vi "Count Itteration.vi"(1 "Reset":bool, 2 "Enable":bool=TRUE, 3 "Direction (Up)":bool=TRUE) -> (4 "Itterations/s":dbl, 7 "Itteration":i32)   [LabVIEW 2012]
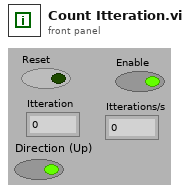
[diagram p1: front panel]
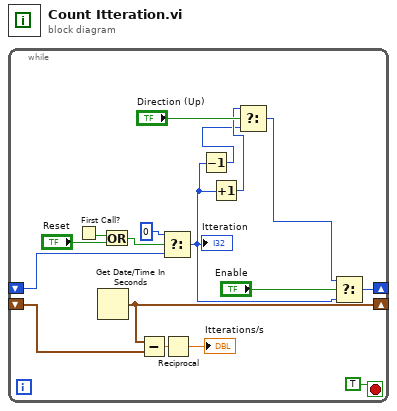
[diagram p0: block diagram]
diagram:
  n1 = while {
    shift-right: [w10] -> _
    shift-left: _ -> [w14]
    shift-right: [w7] -> _
    shift-left: _ -> [w8]
    stop <- TRUE stop-if-true
    n2 = First Call?() -> (First Call?: T/F=w16:bool)
    n3 = Get Date/Time In Seconds() -> (seconds since 1Jan1904=w7:timestamp)
    n4 = Or(x=w16, y="Reset") -> (x .or. y?=w12:bool)
    n5 = Subtract(x=w7, y=w8) -> (x-y=w11:dbl)
    n6 = Select(t=0, s=w12, f=w14) -> (s? t:f=w2:i32)
    "Itteration" <- w2
    n7 = Reciprocal(x=w11) -> (1/x=→"Itterations/s":dbl)
    n8 = Decrement(x=w2) -> (x-1=w1:i32)
    n9 = Increment(x=w2) -> (x+1=w4:i32)
    n10 = Select(t=w4, s="Direction (Up)", f=w1) -> (s? t:f=w3:i32)
    n11 = Select(t=w3, s="Enable", f=w2) -> (s? t:f=w10:i32)
  }
